vi "SetSlide.vi"(8 "error in (no error)":errorcluster, 10 "Number of Steps":i32, 11 "TestBench in":refnum<class "TestBench.lvclass">) -> (0 "error out":errorcluster, 3 "TestBench out":refnum<class "TestBench.lvclass">)   [LabVIEW 2019, in "TestBench.lvlib" / "TestBench.lvclass"]
uses:
  TestBench.lvclass
  TestBench.lvclass/TestBench.ctl
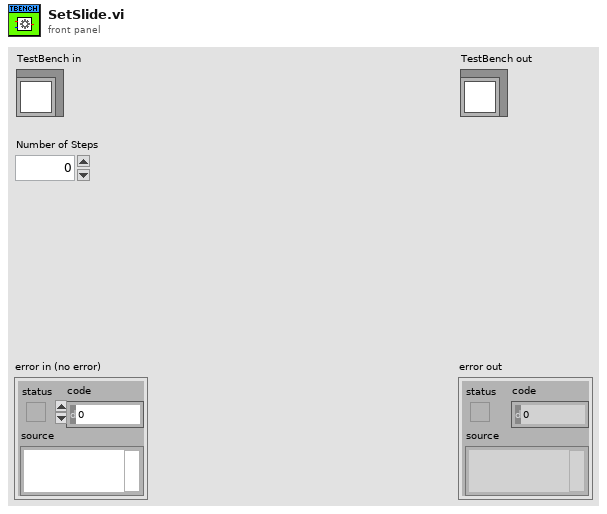
[diagram p1: front panel]
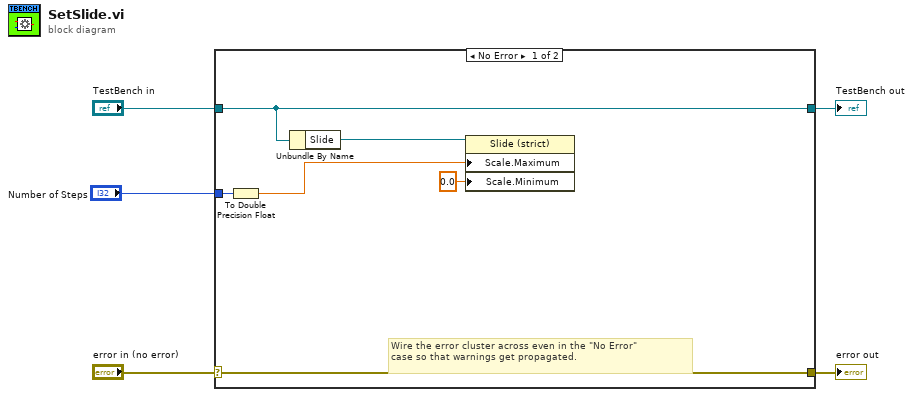
[diagram p0: block diagram]
diagram:
  n1 = case shown="No Error" "error in (no error)" {
    selector: "error in (no error)" -> [w11 w13]
    tunnel: [w11 w13] -> w4
    tunnel: [w10 w12] -> w2
    tunnel: "TestBench in" -> [w10 w12]
    tunnel: "Number of Steps" -> [w8 _]
    frame No Error {
      # "Wire the error cluster across even in the \"No Error\"\ncase so that warnings get propagated."
      n2 = To Double Precision Float(number=w8) -> (double precision float=w7:dbl)
      n3 = Unbundle By Name(w10) -> ("Slide"=w9:refnum<vi>)
      n4 = property class="Slide (strict)"(reference=w9, "Scale.Maximum"=w7, "Scale.Minimum"=0.0 ("Scale.Range:Minimum")) -> ()  [unwired: 1 in, 2 out]
    }
    frame Error {
    }
  }
  "error out" <- w4
  "TestBench out" <- w2
